vi "NotifyIcon - Interpret Event Data.vi"(8 "error in":errorcluster, 10 "NotifyIcon Event Data":variant) -> (0 "error out":errorcluster, 2 "NotifyIcon Event Data":T1)   [LabVIEW 2015]
doc: "Interprets the <b>NotifyIcon Event Data</b> provided by the Event Data terminal of the <NotifyIcon User Event> case of a LabVIEW Event Structure."
uses:
  TypeDefs/NotifyIcon Event Data.ctl
  TypeDefs/NotifyIcon Events.ctl
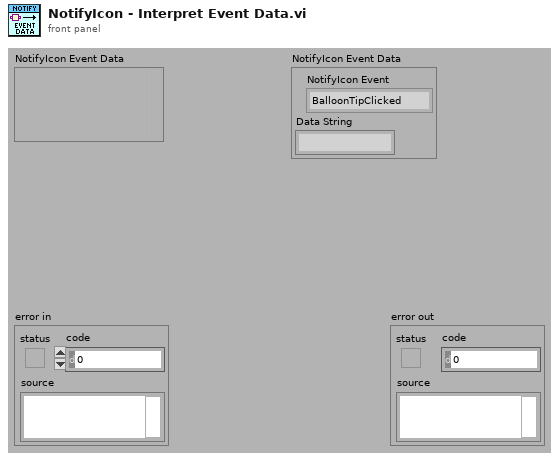
[diagram p1: front panel]
types:
  T1 = typedef "NotifyIcon Event Data.ctl" = cluster{"NotifyIcon Event":T2, "Data String":string}
  T2 = typedef "NotifyIcon Events.ctl" = enum16{"BalloonTipClicked", "BalloonTipClosed", "BalloonTipShown", "Click", "Disposed", "DoubleClick", "MouseClick", "MouseDoubleClick", "MouseDown", "MouseMove", "MouseUp", "MenuItemClick", "MenuItemSelect"}
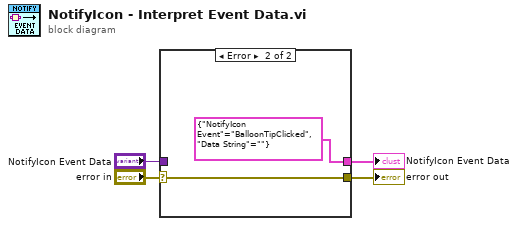
[diagram p0: block diagram]
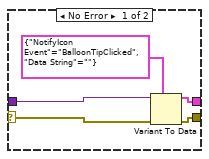
[diagram p2: hidden frame]
diagram:
  n1 = case shown="Error" "error in" {
    selector: "error in" -> [w6 w11]
    tunnel: "NotifyIcon Event Data" -> [w9 _]
    tunnel: [w7 w11] -> w3
    tunnel: [w5 T1 {"NotifyIcon Event"=enum."BalloonTipClicked", "Data String"=""} ("NotifyIcon Event Data")] -> w1
    frame No Error {
      n2 = Variant To Data(error in=w6, type=T1 {"NotifyIcon Event"=enum."BalloonTipClicked", "Data String"=""} ("NotifyIcon Event Data"), Variant=w9) -> (data=w5:T1, error out=w7:errorcluster)
    }
    frame Error {
      (unwired) "" ("Data String")
      (unwired) NotifyIcon_Events."BalloonTipClicked" ("NotifyIcon Events")
    }
  }
  "error out" <- w3
  "NotifyIcon Event Data" <- w1
